vi "alu_one.vi"(2 "C":T1, 3 "S-1":bool, 4 "B":bool, 5 "A":bool) -> (0 "R":bool, 1 "S1":bool)   [LabVIEW 2013]
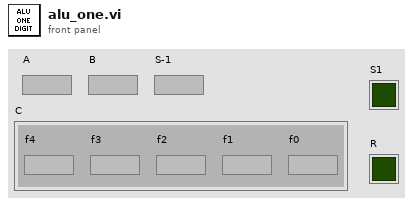
[diagram p1: front panel]
types:
  T1 = cluster{"f4":bool, "f3":bool, "f2":bool, "f1":bool, "f0":bool}
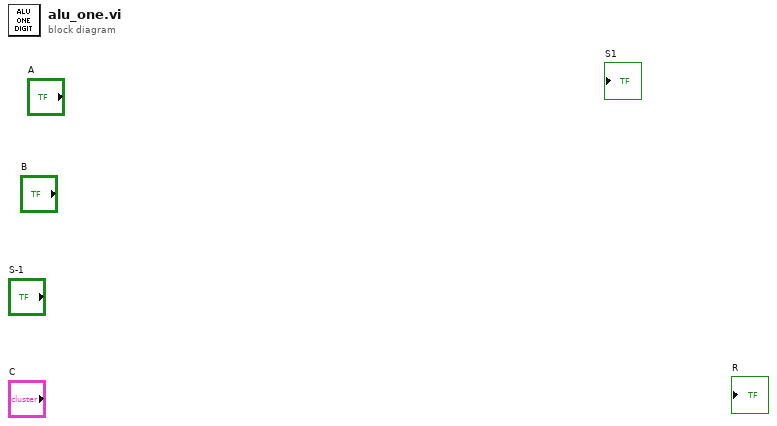
[diagram p0: block diagram]
diagram:
